vi "Compute Protocol Duration.vi"(5 "Protocol":T1[](array[typedef])) -> (1 "Protocol Duration (ms)":dbl[unit], 2 "Protocol Duration (s)":dbl[unit])   [LabVIEW 2019]
uses:
  Controls/Protocol Interval.ctl
  Controls/Stim Interval Mode.ctl
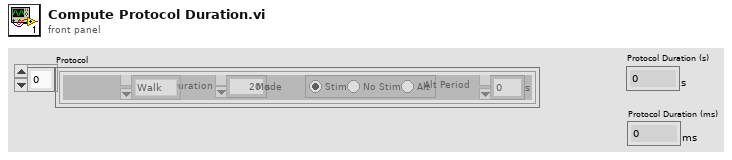
[diagram p1: front panel]
types:
  T1 = typedef "Protocol Interval.ctl" = cluster{"Interval Type":enum16{"Walk", "Rest"}, "Duration":dbl[unit], " Mode":T2, "Alt Period":dbl[unit]}
  T2 = typedef "Stim Interval Mode.ctl" = enum32{"Stim", "No Stim", "Alternating"}
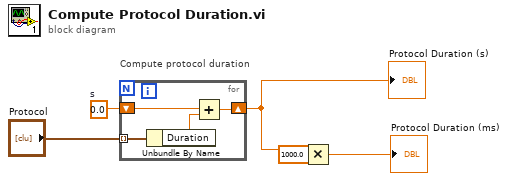
[diagram p0: block diagram]
diagram:
  w4 = dbl[unit] 0.0  # s
  n1 = for "Compute protocol duration" {
    shift-right: [w8] -> w2
    shift-left: w4 -> [w9]
    tunnel: "Protocol" -> [w7] mode=indexing
    n2 = Unbundle By Name(w7) -> ("Duration"=w6:dbl[unit])
    n3 = Add(x=w9, y=w6) -> (x+y=w8:dbl[unit])
  }
  "Protocol Duration (s)" <- w2
  n4 = Multiply(x=w2, y=1000.0) -> (x*y=→"Protocol Duration (ms)":dbl[unit])
